vi "Write Append Numeric.vi"(10 "Append Numeric":u32, 11 "StringIncrementAlgorithm in":refnum<class "StringIncrementAlgorithm.lvclass">) -> (3 "StringIncrementAlgorithm out":refnum<class "StringIncrementAlgorithm.lvclass">)   [LabVIEW 2014, in "UniqueName.lvlib" / "StringIncrementAlgorithm.lvclass"]
uses:
  StringIncrementAlgorithm.lvclass
  StringIncrementAlgorithm.lvclass/StringIncrementAlgorithm.ctl
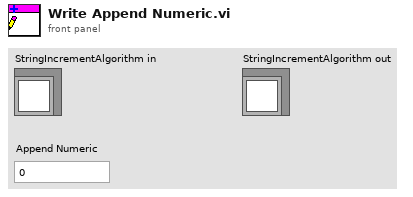
[diagram p1: front panel]
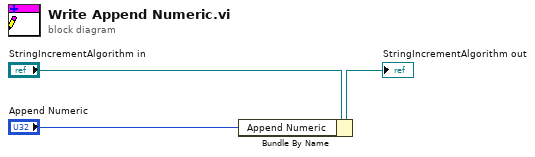
[diagram p0: block diagram]
diagram:
  n1 = Bundle By Name(cluster="StringIncrementAlgorithm in", "Append Numeric"="Append Numeric") -> (→"StringIncrementAlgorithm out":refnum<class "StringIncrementAlgorithm.lvclass">)
